vi "InitDAQmx.vi"(6 "TerminalDirection":tag, 8 "error in (no error)":errorcluster, 9 "CounterStep":tag, 10 "TerminalStep":tag, 11 "StepperController in":refnum<class "StepperController.lvclass">) -> (0 "error out":errorcluster, 3 "StepperController out":refnum<class "StepperController.lvclass">)   [LabVIEW 2013, in "StepperController.lvclass"]
uses:
  StepperController.lvclass
  StepperController.lvclass/StepperController.ctl
  <vilib>/DAQmx/create/channels.llb/DAQmx Create Channel (DO-Digital Output).vi
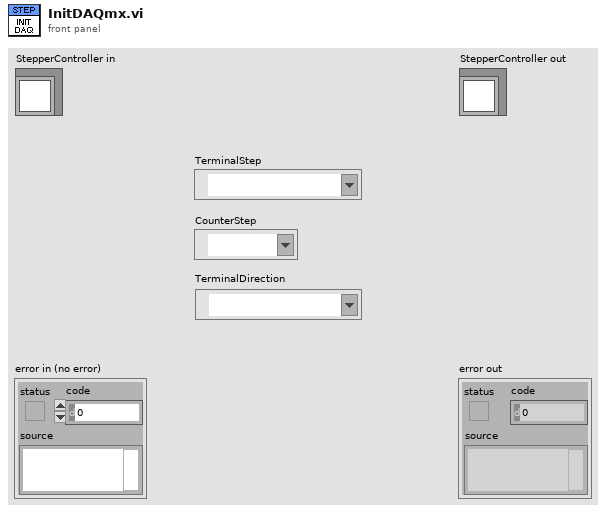
[diagram p1: front panel]
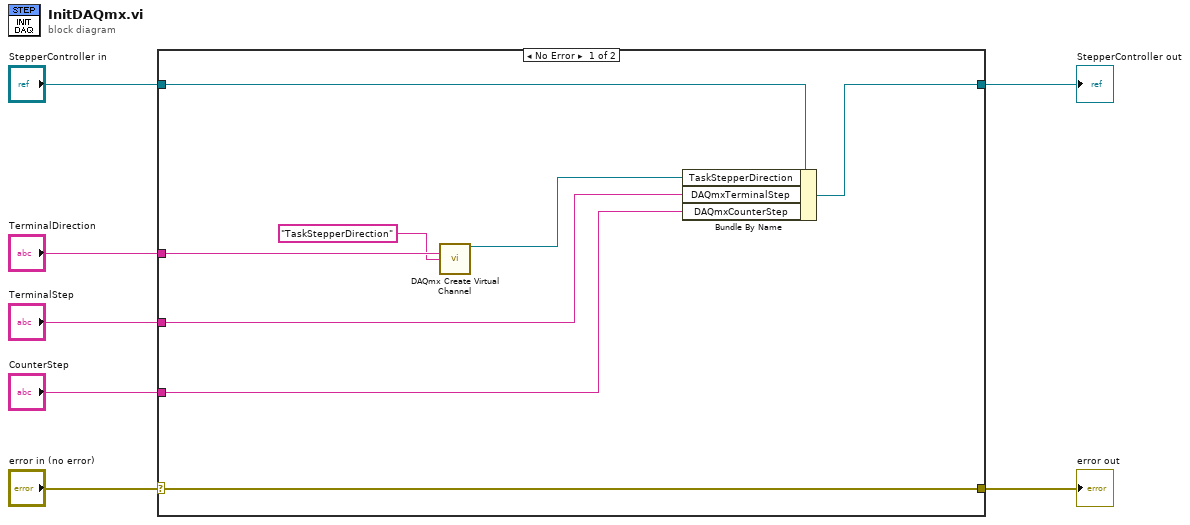
[diagram p0: block diagram]
diagram:
  n1 = case shown="No Error" "error in (no error)" {
    selector: "error in (no error)" -> [w15 w16]
    tunnel: [w15 w16] -> w6
    tunnel: [w13 w17] -> w4
    tunnel: "StepperController in" -> [w14 w17]
    tunnel: "TerminalDirection" -> [w12 _]
    tunnel: "TerminalStep" -> [w8 _]
    tunnel: "CounterStep" -> [w9 _]
    frame No Error {
      n2 = call-poly <vilib>:"DAQmx Create Virtual Channel.vi"("lines"=w12, "name to assign"="TaskStepperDirection") -> ("task out"=w10:refnum<k21>)  [unwired: 12 in, 1 out]
      n3 = Bundle By Name(cluster=w14, "TaskStepperDirection"=w10, "DAQmxTerminalStep"=w8, "DAQmxCounterStep"=w9) -> (w13:refnum<class "StepperController.lvclass">)
    }
    frame Error {
    }
  }
  "error out" <- w6
  "StepperController out" <- w4
